vi "Initialize.vi"(8 "error in":errorcluster, 10 "parameters":variant, 11 "node in":refnum<class "Target.lvclass">) -> (0 "error out":errorcluster, 2 "summary":T2[](array[typedef]), 3 "data value reference":T1)   [LabVIEW 2015, in "Target.lvclass"]
doc: "Initializes the data of a node to its default state.\nThe object is not created inside of this VI, because it is created from a File depending on user selection.\nCopyright 2015 National Instruments Corporation\n\nLicensed under the Apache License, Version 2.0 (the \"License\"); you may not use this file except in compliance with the License. You may obtain a copy of the License at http://www.apache.org/licenses/LICENSE-2.0\nUnless required by applicable law or agreed to in writing, software distributed under the License is distributed on an \"AS IS\" BASIS, WITHOUT WARRANTIES OR CONDITIONS OF ANY KIND, either express or implied. See the License for the specific language governing permissions and limitations under the License."
uses:
  Target.lvclass
  <vilib>/NI/Configuration Framework/Node/Summary.ctl
  <vilib>/NI/Configuration Framework/Node/NodeRef.ctl
  <vilib>/NI/Configuration Framework/Node/NISE_CEF_Node.lvclass
  XML Controls/Supported Targets.ctl
  Target.lvclass/Target.ctl
  VeriStand Custom Device XML Parser.lvlib
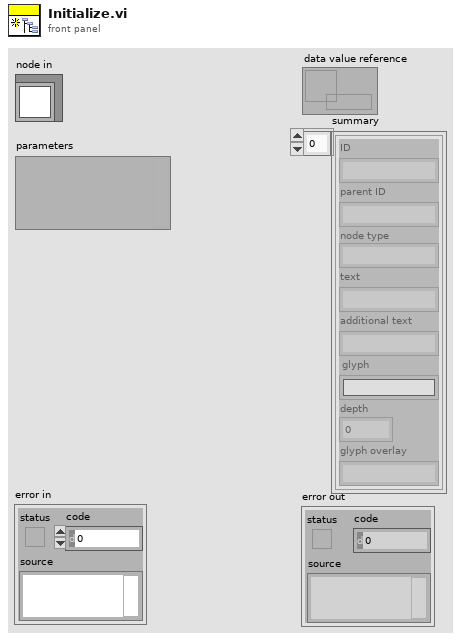
[diagram p1: front panel]
types:
  T1 = typedef "NISE_CEF_Node.lvclass/NodeRef.ctl" = refnum<data-value>
  T2 = typedef "NISE_CEF_Node.lvclass/Summary.ctl" = cluster{"ID":string, "parent ID":string, "node type":string, "text":string, "additional text":string, "glyph":string, "depth":i32, "glyph overlay":string}
  T3 = typedef "VeriStand Custom Device XML Parser.lvlib/Supported Targets.ctl" = enum16{"All", "Pharlap", "VxWorks", "Windows", "Linux_32_ARM", "Linux_x64", "PharlapWindows", "PharlapVxWorks", "VxWorksWindows"}
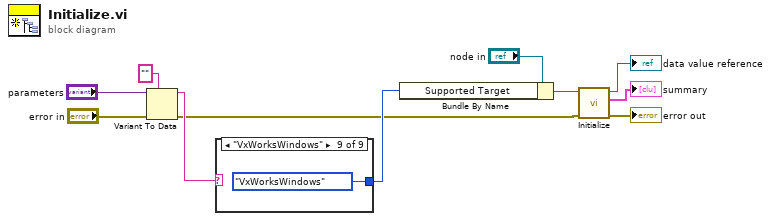
[diagram p0: block diagram]
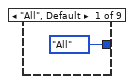
[diagram p2: hidden frame]
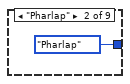
[diagram p3: hidden frame]
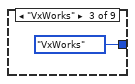
[diagram p4: hidden frame]
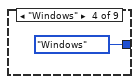
[diagram p5: hidden frame]
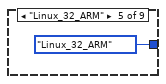
[diagram p6: hidden frame]
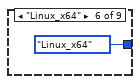
[diagram p7: hidden frame]
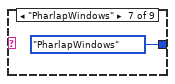
[diagram p8: hidden frame]
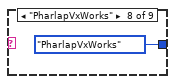
[diagram p9: hidden frame]
diagram:
  n1 = Variant To Data(error in="error in", type="", Variant="parameters") -> (data=w4:string, error out=w1:errorcluster)
  n2 = case shown="\"VxWorksWindows\"" w4 {
    tunnel: [Supported_Targets."All" ("Source.Supported Target") Supported_Targets."Pharlap" ("Source.Supported Target") Supported_Targets."VxWorks" ("Source.Supported Target") Supported_Targets."Windows" ("Source.Supported Target") Supported_Targets."Linux_32_ARM" ("Source.Supported Target") Supported_Targets."Linux_x64" ("Source.Supported Target") Supported_Targets."PharlapWindows" ("Source.Supported Target") Supported_Targets."PharlapVxWorks" ("Source.Supported Target") Supported_Targets."VxWorksWindows" ("Source.Supported Target")] -> w2
    frame "All", Default {
    }
    frame "Pharlap" {
    }
    frame "VxWorks" {
    }
    frame "Windows" {
    }
    frame "Linux_32_ARM" {
    }
    frame "Linux_x64" {
    }
    frame "PharlapWindows" {
    }
    frame "PharlapVxWorks" {
    }
    frame "VxWorksWindows" {
    }
  }
  n3 = Bundle By Name(cluster="node in", "Supported Target"=w2) -> (w3:refnum<class "Target.lvclass">)
  n4 = call-parent "Initialize.vi"("error in"=w1, "node in"=w3) -> ("error out"=→"error out":errorcluster, "summary"=→"summary":T2[], "data value reference"=→"data value reference":T1)  [unwired: 7 in]
